vi "FTW-Actor-Destroy.vi"(0 "FTW Actor Instance":refnum<class "FTW-Actor-Instance.lvclass">, 11 "error in":errorcluster) -> (15 "error out":errorcluster)   [LabVIEW 2015, in "FTW-Actor-Instance.lvclass"]
uses:
  FTW-Actor-Instance.lvclass
  FTW-Actor-Instance.lvclass/FTW-Actor-Instance.ctl
  scheduler/FTW-Scheduler.lvclass
panel:
  # "Inputs"
  # "Outputs"
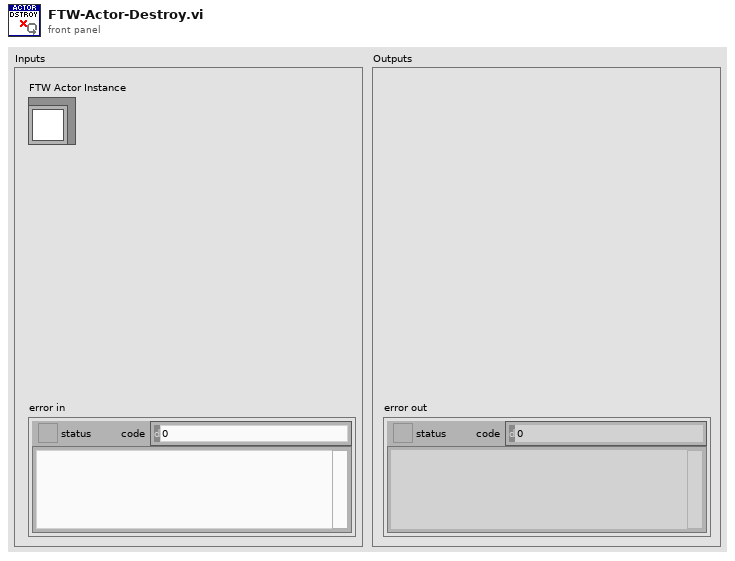
[diagram p1: front panel]
types:
  T1 = typedef "FTW-Type-Actor-Connector.ctl" = refnum<data-value>
  T2 = typedef "FTW-Type-Actor-Inbox.ctl" = refnum<data-value>
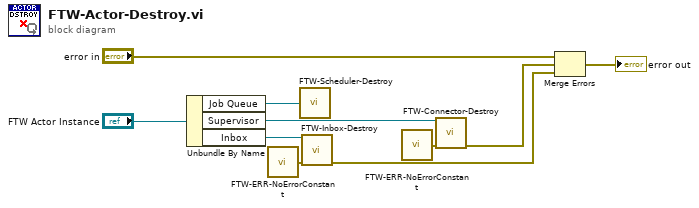
[diagram p0: block diagram]
diagram:
  n1 = Unbundle By Name("FTW Actor Instance") -> ("Job Queue"=w7:refnum<class "FTW-Scheduler.lvclass">, "Supervisor"=w4:T1, "Inbox"=w5:T2)
  n2 = call "FTW-ERR-NoErrorConstant.vi"() -> ("no error"=w2:errorcluster)
  n3 = call "FTW-Scheduler-Destroy.vi"("FTW Job Scheduler"=w7) -> ()  [unwired: 1 out]
  n4 = call "FTW-Inbox-Destroy.vi"("FTW Inbox"=w5, "error in"=w2) -> ("error out"=w6:errorcluster)  [unwired: 13 in]
  n5 = call "FTW-ERR-NoErrorConstant.vi"() -> ("no error"=w1:errorcluster)
  n6 = call "FTW-Connector-Destroy.vi"("FTW Actor Connector"=w4, "error in"=w1) -> ("error out"=w3:errorcluster)  [unwired: 13 in]
  n7 = Merge Errors("error in", w3, w6) -> (→"error out":errorcluster)
